vi "Deg - Rad.vi"(1 "Degrees IN":dbl) -> (0 "Radian OUT":dbl)   [LabVIEW 2019]
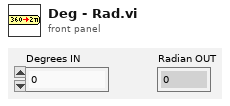
[diagram p1: front panel]
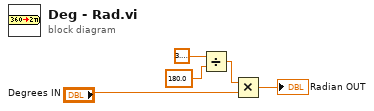
[diagram p0: block diagram]
diagram:
  n1 = Divide(x=3.141592653589793, y=180.0) -> (x/y=w5:dbl)
  n2 = Multiply(x=w5, y="Degrees IN") -> (x*y=→"Radian OUT":dbl)
